vi "Build Full Name.vi"(10 "Index":i32, 11 "Item Graph In":T1[](array[typedef])) -> (2 "Name":string, 3 "Item Graph":T1[](array[typedef]))   [LabVIEW 2020, in "Better Search.lvlib"]
uses:
  Better Search.lvlib
  Data Types/Type Reflection Item.ctl
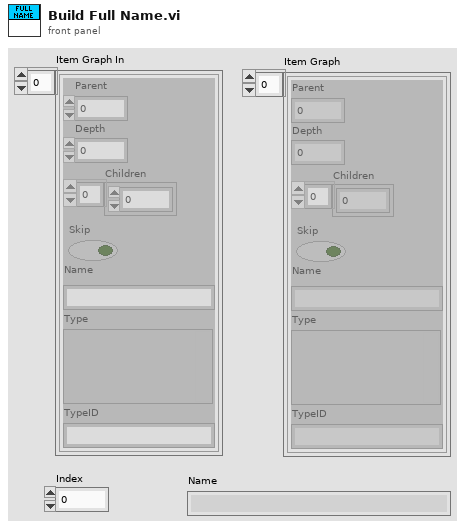
[diagram p1: front panel]
types:
  T1 = typedef "Better Search.lvlib/Type Reflection Item.ctl" = cluster{"Parent":i32, "Depth":i32, "Children":i32[], "Skip":bool, "Name":string, "Type":variant, "TypeID":string}
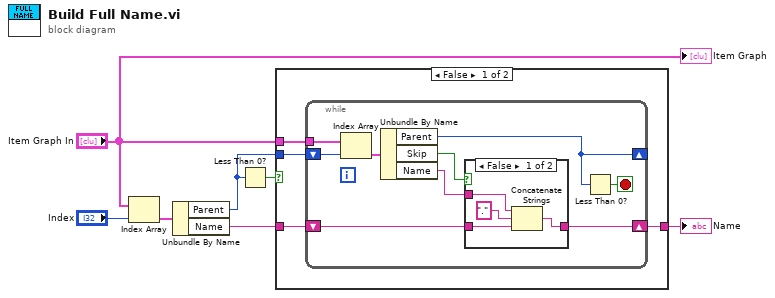
[diagram p0: block diagram]
diagram:
  n1 = Index Array(array="Item Graph In", index="Index") -> (element=w4:T1)
  n2 = Unbundle By Name(w4) -> ("Parent"=w2:i32, "Name"=w3:string)
  n3 = Less Than 0?(x=w2) -> (x < 0?=w1:bool)
  n4 = case shown="False" w1 {
    tunnel: w3 -> [w10 w26]
    tunnel: [w9 w26] -> w7
    tunnel: "Item Graph In" -> [w8 _]
    tunnel: w2 -> [w11 _]
    frame False {
      n5 = while {
        shift-right: [w17] -> _
        shift-left: w11 -> [w14]
        shift-right: [w15] -> w9
        shift-left: w10 -> [w16]
        tunnel: w8 -> [w19]
        stop <- w20 stop-if-true
        n6 = Index Array(array=w19, index=w14) -> (element=w18:T1)
        n7 = Unbundle By Name(w18) -> ("Parent"=w17:i32, "Skip"=w12:bool, "Name"=w13:string)
        n8 = case shown="False" w12 {
          tunnel: w16 -> [w24 w25]
          tunnel: w13 -> [w23 _]
          tunnel: [w21 w25] -> w15
          frame False {
            n9 = Concatenate Strings(w23, "." ("string"), w24) -> (w21:string)
          }
          frame True {
          }
        }
        n10 = Less Than 0?(x=w17) -> (x < 0?=w20:bool)
      }
    }
    frame True {
    }
  }
  "Name" <- w7
  "Item Graph" <- "Item Graph In"
